vi "LogFilePath.vi"(8 "error in (no error)":errorcluster) -> (0 "error out":errorcluster, 3 "appended path":path)   [LabVIEW 2019]
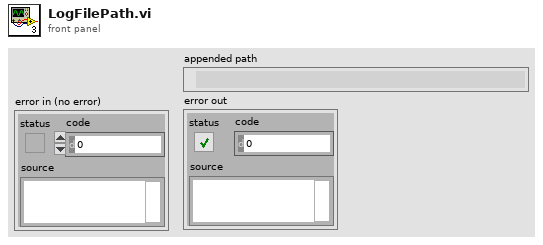
[diagram p1: front panel]
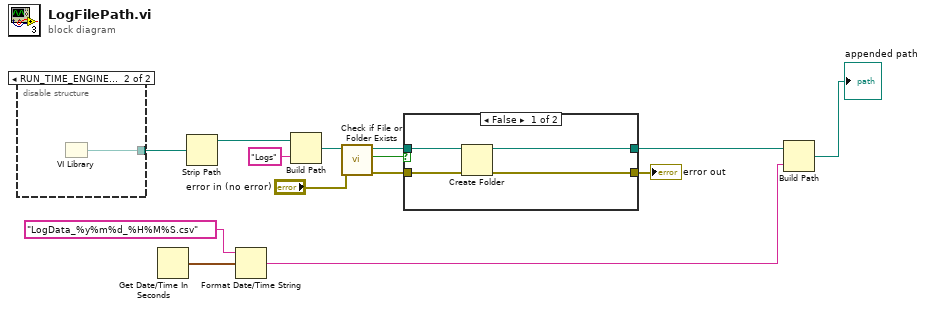
[diagram p0: block diagram]
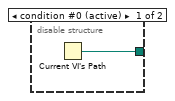
[diagram p3: hidden frame]
diagram:
  n1 = disable-structure shown="RUN_TIME_ENGINE==True" {
    disable-tunnel: [w15 w16] -> w14
    frame condition #0 (active) {
      n2 = Current VI's Path() -> (path=w15:path)
    }
    frame condition #1 {
      n3 = VI Library() -> (path=w16:path)
    }
  }
  n4 = Get Date/Time In Seconds() -> (seconds since 1Jan1904=w11:timestamp)
  n5 = Strip Path(path=w14) -> (stripped path=w13:path)  [unwired: 1 out]
  n6 = Format Date/Time String(time format string (%c)="LogData_%y%m%d_%H%M%S.csv", seconds (now)=w11) -> (date/time string=w9:string)  [unwired: 1 in]
  n7 = Build Path(base path=w13, name or relative path="Logs") -> (appended path=w7:path)
  n8 = call <vilib>:"Check if File or Folder Exists.vi"("error in (no error)"="error in (no error)", "path"=w7) -> ("error out"=w4:errorcluster, "file or folder exists?"=w6:bool, "dup path"=w5:path)  [unwired: 7 in]
  n9 = case shown="False" w6 {
    tunnel: w5 -> [w20 w22]
    tunnel: w4 -> [w19 w21]
    tunnel: [w18 w21] -> w1
    tunnel: [w17 w22] -> w3
    frame False {
      n10 = Create Folder(path (use dialog)=w20, error in=w19) -> (created path=w17:path, error out=w18:errorcluster)  [unwired: 1 in, 1 out]
    }
    frame True {
    }
  }
  "error out" <- w1
  n11 = Build Path(base path=w3, name or relative path=w9) -> (appended path=→"appended path":path)
